vi "Scanner_Mirror_configuration.vi"(0 "POS X":dbl, 1 "POS Y":dbl, 2 "POS Z":dbl, 5 "error in":errorcluster) -> (19 "error out":errorcluster)   [LabVIEW 2013]
uses:
  Utilities/controls/ctlSeqFNs_PI_SysNr.ctl
  Variables/GlobalSetConfigurationPhysikalInstruments.vi
  Variables/GlobalSetNumberOfDigits_Scanners.vi
  Variables/GlobalSetGetPositionParameters.vi
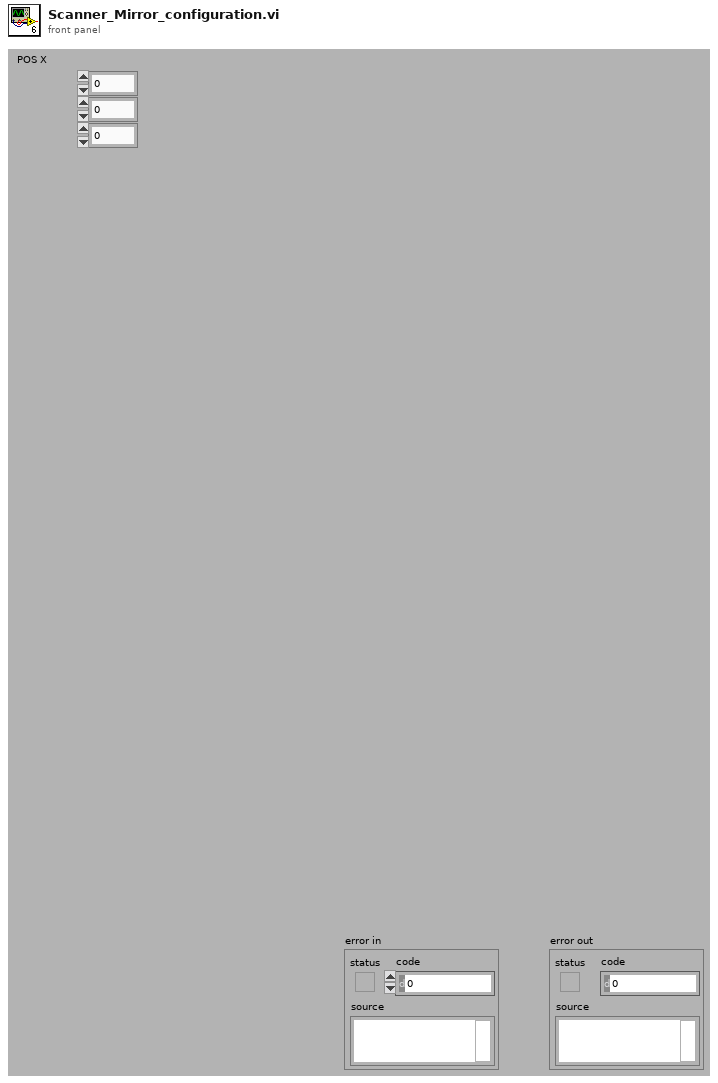
[diagram p1: front panel]
types:
  T1 = typedef "ctlSeqFNs_PI_SysNr.ctl" = enum16{"Zero", "E517", "E710"}
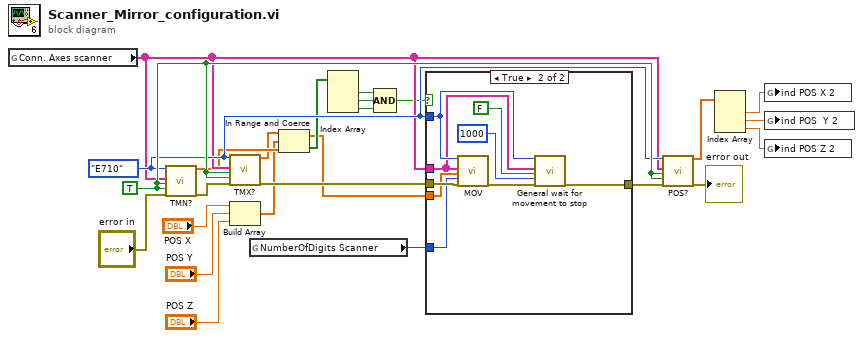
[diagram p0: block diagram]
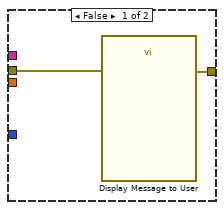
[diagram p2: hidden frame]
diagram:
  w18 = ctlSeqFNs_PI_SysNr."E710" ("DeviceNr.")
  w24 = TRUE ("All axes?")
  n1 = global read "GlobalSetConfigurationPhysikalInstruments.vi" "Conn. Axes scanner"() -> (w17:string[])
  n2 = call "TMN?.vi"("System no."=w18, "Axes to query"=w17, "All axes?"=w24, "Axis identifier?"=w24, "error in"="error in") -> ("Minimum travel limit"=w12:dbl[], "error out"=w23:errorcluster)  [unwired: 13 in]
  n3 = call "TMX?.vi"("System no."=w18, "Axes to query"=w17, "All axes?"=w24, "Axis identifier?"=w24, "error in"=w23) -> ("Maximum travel limit"=w11:dbl[], "error out"=w25:errorcluster)  [unwired: 13 in]
  n4 = Build Array("POS X", "POS Y", "POS Z") -> (w10:dbl[])
  n5 = global read "GlobalSetNumberOfDigits_Scanners.vi" "NumberOfDigits Scanner"() -> (w21:i32)
  n6 = In Range and Coerce(upper limit=w11, x=w10, lower limit=w12) -> (coerced(x)=w9:dbl[], In Range?=w16:bool[])
  n7 = Index Array(array=w16) -> (element #1=w15:bool, element #2=w14:bool, element #3=w13:bool)  [unwired: 3 in]
  n8 = Compound Arithmetic op=AND(w15, w14, w13) -> (w8:bool)
  n9 = case shown="True" w8 {
    tunnel: w25 -> [w26 w36]
    tunnel: w21 -> [_ w35]
    tunnel: [w27 w31] -> w19
    tunnel: w18 -> [_ w30]
    tunnel: w17 -> [_ w29]
    tunnel: w9 -> [_ w28]
    frame False {
      n10 = call "Display Message to User"("error in (no error)"=w26) -> ("error out"=w27:errorcluster)  [unwired: 9 in, 1 out]
    }
    frame True {
      n11 = call "MOV.vi"("System no."=w30, "Axes to move"=w29, "Position values"=w28, "No.of digits"=w35, "error in"=w36) -> ("error out"=w32:errorcluster)  [unwired: 14 in]
      n12 = call "General wait for movement to stop.vi"("System no."=w30, "Axes to wait for"=w29, "All axes?"=FALSE, "Additional wait time, ms"=u32 1000, "error in"=w32) -> ("error out"=w31:errorcluster)  [unwired: 13 in, 1 out]
    }
  }
  n13 = call "POS?.vi"("System no."=w18, "Axes to query"=w17, "All axes?"=w24, "Axis identifier?"=w24, "error in"=w19) -> ("Position"=w7:dbl[], "error out"=→"error out":errorcluster)  [unwired: 13 in]
  n14 = Index Array(array=w7) -> (element #1=w6:dbl, element #2=w5:dbl, element #3=w4:dbl)  [unwired: 3 in]
  n15 = global write "GlobalSetGetPositionParameters.vi" "ind POS X 2"(w6) -> ()
  n16 = global write "GlobalSetGetPositionParameters.vi" "ind POS  Y 2"(w5) -> ()
  n17 = global write "GlobalSetGetPositionParameters.vi" "ind POS Z 2"(w4) -> ()
